vi "Assert XML Project.vi"() -> ()   [LabVIEW 2015, in "XML Project.lvclass"]
uses:
  XML Project.lvclass
  Brower Console/Models/BrowerComponent/BrowerComposite/protected/ObjectAttributes.ctl
  Brower Console/Models/BrowerComponent/BrowerComponent/BrowerComponent.lvclass
  Brower Console/Models/BrowerComponent/BrowerComposite/BrowerComposite.lvclass
  Brower Console/Models/BrowerComponent/BrowerLeaf/BrowerLeaf.lvclass
  <vilib>/NI/AQ Character Lineator/JSON Serializer/JSON Serializer.lvclass
  <vilib>/NI/AQ Character Lineator/Serializer/Serializer.lvclass
  <vilib>/NI/AQ Character Lineator/Deserializer/Deserializer.lvclass
  <vilib>/NI/AQ Character Lineator/JSON Deserializer/JSON Deserializer.lvclass
panel:
  out "SymbolIndex":i32
  out "ComponentName 2":string
  in  "XML File Path":path
  out "ComponentName":string
  out "data":T1
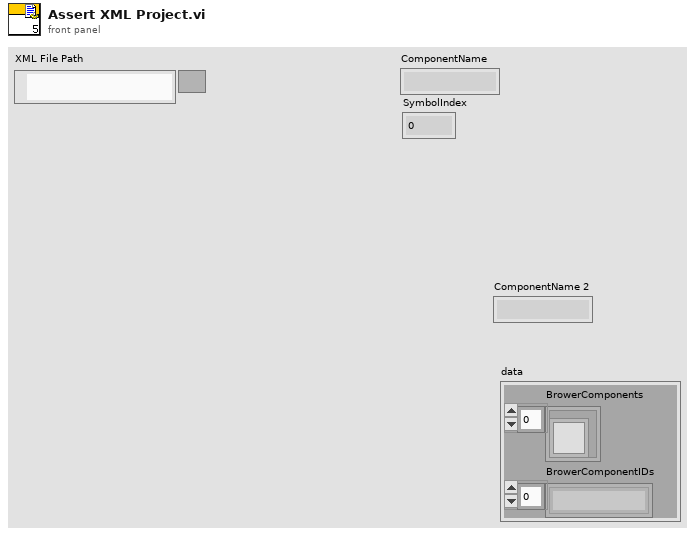
[diagram p1: front panel]
types:
  T1 = typedef "BrowerComposite.lvclass/ObjectAttributes.ctl" = cluster{"BrowerComponents":refnum<class "BrowerComponent.lvclass">[], "BrowerComponentIDs":string[]}
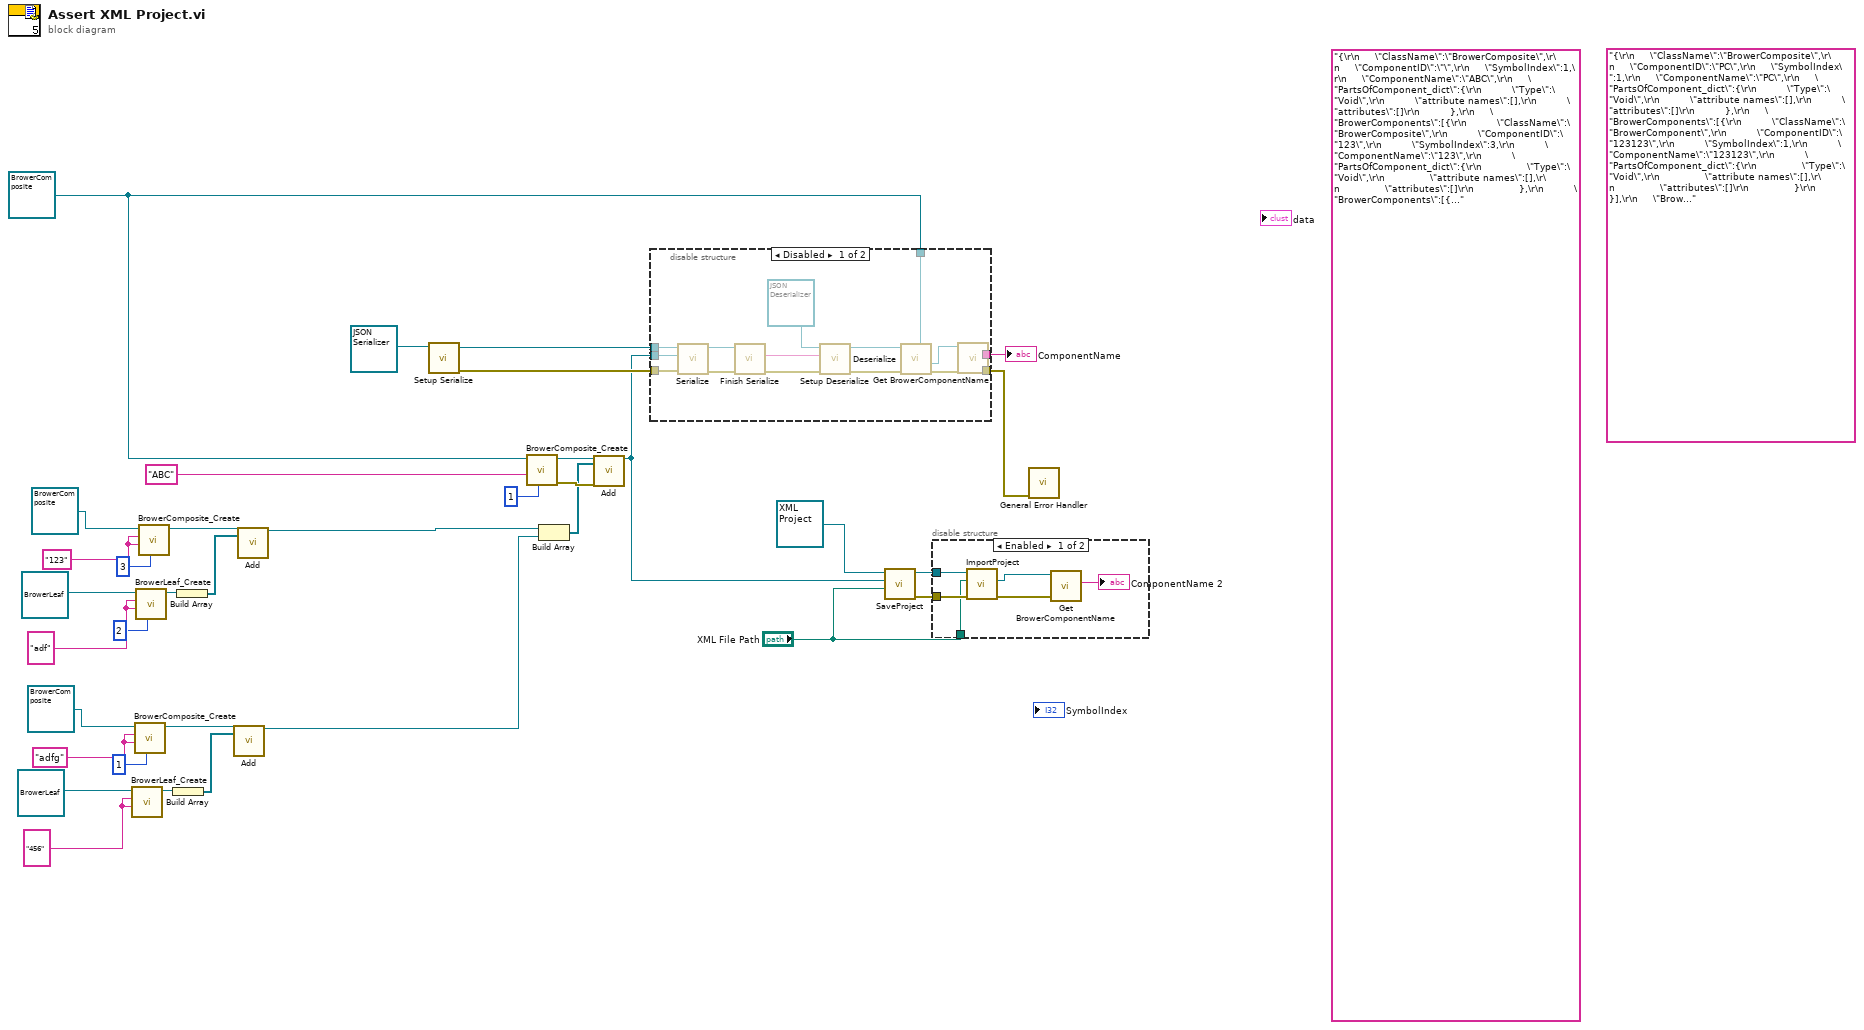
[diagram p0: block diagram]
diagram:
  (unwired) "{\r\n     \"ClassName\":\"BrowerComposite\",\r\n     \"ComponentID\":\"PC\",\r\n     \"SymbolIndex\":1,\r\n     \"ComponentName\":\"PC\",\r\n     \"PartsOfComponent_dict\":{\r\n          \"Type\":\"Void\",\r\n          \"attribute names\":[],\r\n          \"attributes\":[]\r\n          },\r\n     \"BrowerComponents\":[{\r\n          \"ClassName\":\"BrowerComponent\",\r\n          \"ComponentID\":\"123123\",\r\n          \"SymbolIndex\":1,\r\n          \"ComponentName\":\"123123\",\r\n          \"PartsOfComponent_dict\":{\r\n               \"Type\":\"Void\",\r\n               \"attribute names\":[],\r\n               \"attributes\":[]\r\n               }\r\n          }],\r\n     \"BrowerComponentIDs\":[\"123123\"]\r\n     }" ("String")
  (unwired) "{\r\n     \"ClassName\":\"BrowerComposite\",\r\n     \"ComponentID\":\"\",\r\n     \"SymbolIndex\":1,\r\n     \"ComponentName\":\"ABC\",\r\n     \"PartsOfComponent_dict\":{\r\n          \"Type\":\"Void\",\r\n          \"attribute names\":[],\r\n          \"attributes\":[]\r\n          },\r\n     \"BrowerComponents\":[{\r\n          \"ClassName\":\"BrowerComposite\",\r\n          \"ComponentID\":\"123\",\r\n          \"SymbolIndex\":3,\r\n          \"ComponentName\":\"123\",\r\n          \"PartsOfComponent_dict\":{\r\n               \"Type\":\"Void\",\r\n               \"attribute names\":[],\r\n               \"attributes\":[]\r\n               },\r\n          \"BrowerComponents\":[{\r\n               \"ClassName\":\"BrowerLeaf\",\r\n               \"ComponentID\":\"adf\",\r\n               \"SymbolIndex\":2,\r\n               \"ComponentName\":\"adf\",\r\n               \"PartsOfComponent_dict\":{\r\n                    \"Type\":\"Void\",\r\n                    \"attribute names\":[],\r\n                    \"attributes\":[]\r\n                    }\r\n               }],\r\n          \"BrowerComponentIDs\":[\"adf\"]\r\n          },{\r\n          \"ClassName\":\"BrowerComposite\",\r\n          \"ComponentID\":\"adfg\",\r\n          \"SymbolIndex\":1,\r\n          \"ComponentName\":\"adfg\",\r\n          \"PartsOfComponent_dict\":{\r\n               \"Type\":\"Void\",\r\n               \"attribute names\":[],\r\n               \"attributes\":[]\r\n               },\r\n          \"BrowerComponents\":[{\r\n               \"ClassName\":\"BrowerLeaf\",\r\n               \"ComponentID\":\"456\",\r\n               \"SymbolIndex\":0,\r\n               \"ComponentName\":\"456\",\r\n               \"PartsOfComponent_dict\":{\r\n                    \"Type\":\"Void\",\r\n                    \"attribute names\":[],\r\n                    \"attributes\":[]\r\n                    }\r\n               }],\r\n          \"BrowerComponentIDs\":[\"456\"]\r\n          }],\r\n     \"BrowerComponentIDs\":[\"123\",\"adfg\"]\r\n     }" ("String")
  w23 = "456" ("ComponentID")
  w22 = "adfg" ("ComponentName")
  w26 = "adf" ("ComponentID")
  w27 = "123" ("ComponentName")
  w12 = refnum<class "BrowerComposite.lvclass"> refnum ("BrowerComposite")
  n1 = call "BrowerLeaf_Create.vi"("ComponentName"=w23, "ComponentID"=w23, "reference in"=refnum<class "BrowerLeaf.lvclass"> refnum ("BrowerLeaf")) -> ("reference out"=w21:refnum<class "BrowerLeaf.lvclass">)  [unwired: 7 in, 1 out]
  n2 = call "BrowerComposite_Create.vi"("SymbolIndex"=1, "ComponentName"=w22, "ComponentID"=w22, "reference in"=refnum<class "BrowerComposite.lvclass"> refnum ("BrowerComposite")) -> ("reference out"=w20:refnum<class "BrowerComposite.lvclass">)  [unwired: 6 in, 1 out]
  n3 = call "BrowerLeaf_Create.vi"("SymbolIndex"=2, "ComponentName"=w26, "ComponentID"=w26, "reference in"=refnum<class "BrowerLeaf.lvclass"> refnum ("BrowerLeaf")) -> ("reference out"=w29:refnum<class "BrowerLeaf.lvclass">)  [unwired: 6 in, 1 out]
  n4 = call "BrowerComposite_Create.vi"("SymbolIndex"=3, "ComponentName"=w27, "ComponentID"=w27, "reference in"=refnum<class "BrowerComposite.lvclass"> refnum ("BrowerComposite")) -> ("reference out"=w30:refnum<class "BrowerComposite.lvclass">)  [unwired: 6 in, 1 out]
  n5 = Build Array(w21) -> (w24:refnum<class "BrowerLeaf.lvclass">[])
  n6 = Build Array(w29) -> (w25:refnum<class "BrowerLeaf.lvclass">[])
  n7 = call-dynamic "Add.vi"("reference in"=w20, "BrowerComponents"=w24) -> ("reference out"=w17:refnum<class "BrowerComposite.lvclass">)  [unwired: 16 in, 1 out]
  n8 = call-dynamic "Add.vi"("reference in"=w30, "BrowerComponents"=w25) -> ("reference out"=w28:refnum<class "BrowerComposite.lvclass">)  [unwired: 16 in, 1 out]
  n9 = call <vilib>:"Setup Serialize.vi"("Serializer in"=refnum<class "JSON Serializer.lvclass"> refnum ("JSON Serializer.lvclass")) -> ("error out"=w14:errorcluster, "Serializer out"=w13:refnum<class "JSON Serializer.lvclass">)  [unwired: 9 in]
  n10 = call "BrowerComposite_Create.vi"("SymbolIndex"=1, "ComponentName"="ABC", "reference in"=w12) -> ("error out"=w35:errorcluster, "reference out"=w34:refnum<class "BrowerComposite.lvclass">)  [unwired: 7 in]
  n11 = Build Array(w28, w17) -> (w33:refnum<class "BrowerComposite.lvclass">[])
  n12 = call-dynamic "Add.vi"("reference in"=w34, "BrowerComponents"=w33, "error in (no error)"=w35) -> ("reference out"=w9:refnum<class "BrowerComposite.lvclass">)  [unwired: 15 in, 1 out]
  n13 = disable-structure shown="Disabled" {
    disable-tunnel: w14 -> [w50 _]
    disable-tunnel: w13 -> [w49 _]
    disable-tunnel: w12 -> [w43 _]
    disable-tunnel: [w40 _] -> w11
    disable-tunnel: [w39 _] -> w10
    disable-tunnel: w9 -> [w36 _]
    frame Disabled {
      n14 = call-dynamic "Serialize.vi"("error in (no error)"=w50, "Serializable"=w36, "JSON Serializer in"=w49) -> ("error out"=w47:errorcluster, "JSON Serializer out"=w48:refnum<class "JSON Serializer.lvclass">)  [unwired: 7 in]
      n15 = call <vilib>:"Finish Serialize.vi"("error in (no error)"=w47, "Serializer in"=w48) -> ("error out"=w38:errorcluster, "String"=w46:string)  [unwired: 6 in, 2 out]
      n16 = call <vilib>:"Setup Deserialize.vi"("error in (no error)"=w38, "String"=w46, "Deserializer in"=refnum<class "JSON Deserializer.lvclass"> refnum ("JSON Deserializer.lvclass")) -> ("error out"=w44:errorcluster, "Deserializer out"=w45:refnum<class "JSON Deserializer.lvclass">)  [unwired: 7 in]
      n17 = call <vilib>:"Deserialize.vi"("Target Type (Serializable.lvclass)"=w43, "error in (no error)"=w44, "Deserializer in"=w45) -> ("error out"=w41:errorcluster, "Serializable"=w42:refnum<class "BrowerComposite.lvclass">)  [unwired: 5 in, 2 out]
      n18 = call "Get BrowerComponentName.vi"("error in (no error)"=w41, "BrowerComponent in"=w42) -> ("error out"=w39:errorcluster, "ComponentName"=w40:string)  [unwired: 7 in, 1 out]
    }
    frame Enabled {
    }
  }
  "ComponentName" <- w11
  n19 = call "SaveProject.vi"("XML File Path"="XML File Path", "BrowerComponent"=w9, "XML Project"=refnum<class "XML Project.lvclass"> refnum) -> ("error out"=w6:errorcluster, "ProjectManager out"=w7:refnum<class "XML Project.lvclass">)  [unwired: 7 in]
  n20 = disable-structure shown="Enabled" {
    disable-tunnel: w7 -> [w56 _]
    disable-tunnel: w6 -> [w55 _]
    disable-tunnel: "XML File Path" -> [w54 _]
    frame Enabled {
      n21 = call "ImportProject.vi"("error in (no error)"=w55, "XML File Path"=w54, "ProjectManager in"=w56) -> ("error out"=w51:errorcluster, "value"=w52:refnum<class "BrowerComponent.lvclass">)  [unwired: 6 in, 1 out]
      n22 = call "Get BrowerComponentName.vi"("error in (no error)"=w51, "BrowerComponent in"=w52) -> ("ComponentName"=→"ComponentName 2":string)  [unwired: 7 in, 2 out]
    }
    frame Disabled {
    }
  }
  n23 = call <vilib>:"General Error Handler.vi"("error in (no error)"=w10) -> ()  [unwired: 10 in, 5 out]
